vi "Add Icon From Picture.vi"(7 "Icon Index (Next)":i32=-1, 8 "error in (no error)":errorcluster, 9 "Icon Name":string, 10 "Picture":picture, 11 "Toolbar Control in":refnum<class "Toolbar Control.lvclass">) -> (0 "error out":errorcluster, 3 "Toolbar Control out":refnum<class "Toolbar Control.lvclass">)   [LabVIEW 2011, in "Toolbar Control.lvclass"]
doc: "This VI will add the image <B>Picture</B> to the <B>Toolbar Control in</B> at the available location or if specified by <B>Icon Index (Next)</B>. The name of the icon is specified by <B>Icon Name</B>.\n\n-------------\nDeveloped by Brian Hoover (hooovahh)"
uses:
  Toolbar Control.lvclass
  Toolbar Control.lvclass/Toolbar Control.ctl
  Controls/Icon Data.ctl
  <vilib>/picture/picture.llb/imagedata.ctl
  Controls/Button State.ctl
  Controls/Icon Type.ctl
  <vilib>/Utility/miscctls.llb/LVRectTypeDef.ctl
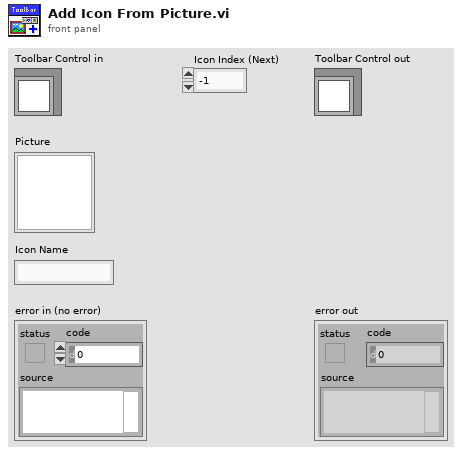
[diagram p1: front panel]
types:
  T1 = typedef "LVRectTypeDef.ctl" = cluster{"Left":i16, "Top":i16, "Right":i16, "Bottom":i16}
  T2 = typedef "Toolbar Control.lvclass/Icon Data.ctl" = cluster{"Original Image Path":path, "Original Image Data":T3, "Scaled Icon":picture, "Button Name":string, "Button State":T4, "Icon Type":T5}
  T3 = typedef "imagedata.ctl" = cluster{"image type":i32, "image depth":i32, "image":u8[], "mask":u8[], "colors":u32[], "Rectangle":cluster{"left":i16, "top":i16, "right":i16, "bottom":i16}}
  T4 = typedef "Toolbar Control.lvclass/Button State.ctl" = enum8{"Enabled", "Disabled", "Disabled and Grayed Out"}
  T5 = typedef "Icon Type.ctl" = enum16{"Normal Icon", "Separator Icon", "More Options"}
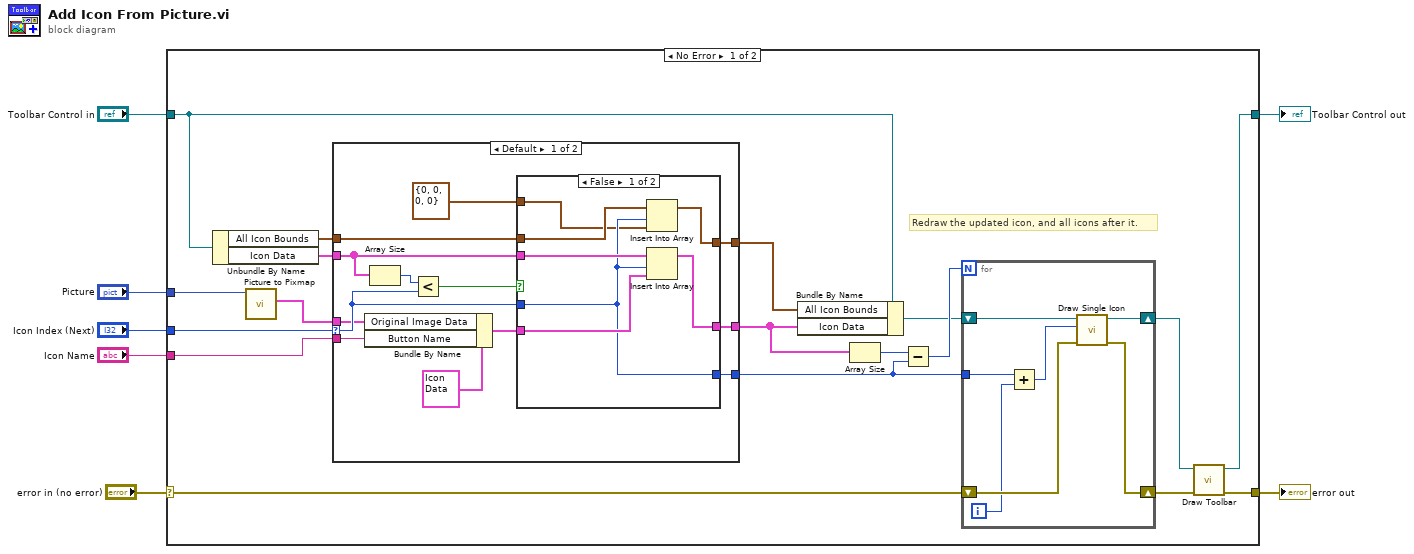
[diagram p0: block diagram]
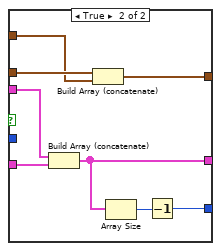
[diagram p2: hidden frame]
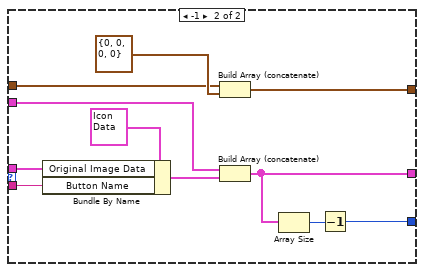
[diagram p3: hidden frame]
diagram:
  n1 = case shown="No Error" "error in (no error)" {
    selector: "error in (no error)" -> [w12 w73]
    tunnel: [w8 w73] -> w6
    tunnel: [w9 w72] -> w4
    tunnel: "Toolbar Control in" -> [w25 w72]
    tunnel: "Picture" -> [w21 _]
    tunnel: "Icon Index (Next)" -> [w23 _]
    tunnel: "Icon Name" -> [w22 _]
    frame No Error {
      # "Redraw the updated icon, and all icons after it."
      n2 = Unbundle By Name(w25) -> ("All Icon Bounds"=w19:T1[], "Icon Data"=w24:T2[])
      n3 = call <vilib>:"Picture to Pixmap.vi"("picture"=w21) -> ("image data"=w20:T3)  [unwired: 9 in, 1 out]
      n4 = case shown="Default" w23 {
        selector: w23 -> [w38 _]
        tunnel: w20 -> [w37 w70]
        tunnel: w22 -> [w45 w69]
        tunnel: w24 -> [w43 w68]
        tunnel: [w39 w65] -> w14
        tunnel: [w36 w64] -> w15
        tunnel: w19 -> [w35 w62]
        tunnel: [w34 w61] -> w18
        frame Default {
          n5 = Bundle By Name(cluster=T2 {"Original Image Path"=path "", "Original Image Data"={"image type"=0, "image depth"=0, "image"=[], "mask"=[], "colors"=[], "Rectangle"={"left"=0, "top"=0, "right"=0, "bottom"=0}}, "Scaled Icon"=bytes[0], "Button Name"="", "Button State"=enum."Enabled", "Icon Type"=enum."Normal Icon"} ("Cluster"), "Original Image Data"=w37, "Button Name"=w45) -> (w40:T2)
          n6 = Array Size(array=w43) -> (size(s)=w42:i32)
          n7 = Less?(x=w42, y=w38) -> (x < y?=w41:bool)
          n8 = case shown="False" w41 {
            tunnel: w43 -> [w52 w60]
            tunnel: w40 -> [w51 w59]
            tunnel: [w50 w57] -> w39
            tunnel: w38 -> [w47 _]
            tunnel: [w47 w56] -> w36
            tunnel: w35 -> [w48 w55]
            tunnel: [w49 w54] -> w34
            tunnel: T1 {"Left"=0, "Top"=0, "Right"=0, "Bottom"=0} ("Icon Bounds") -> [w46 w53]
            frame False {
              n9 = Insert Into Array(array=w48, index=w47, new element=w46) -> (w49:T1[])
              n10 = Insert Into Array(array=w52, index=w47, new element=w51) -> (w50:T2[])
            }
            frame True {
              n11 = Build Array (concatenate)(w60, w59) -> (w57:T2[])
              n12 = Build Array (concatenate)(w55, w53) -> (w54:T1[])
              n13 = Array Size(array=w57) -> (size(s)=w58:i32)
              n14 = Decrement(x=w58) -> (x-1=w56:i32)
            }
          }
        }
        frame -1 {
          n15 = Bundle By Name(cluster=T2 {"Original Image Path"=path "", "Original Image Data"={"image type"=0, "image depth"=0, "image"=[], "mask"=[], "colors"=[], "Rectangle"={"left"=0, "top"=0, "right"=0, "bottom"=0}}, "Scaled Icon"=bytes[0], "Button Name"="", "Button State"=enum."Enabled", "Icon Type"=enum."Normal Icon"} ("Cluster"), "Original Image Data"=w70, "Button Name"=w69) -> (w67:T2)
          n16 = Build Array (concatenate)(w62, T1 {"Left"=0, "Top"=0, "Right"=0, "Bottom"=0} ("Icon Bounds")) -> (w61:T1[])
          n17 = Build Array (concatenate)(w68, w67) -> (w65:T2[])
          n18 = Array Size(array=w65) -> (size(s)=w66:i32)
          n19 = Decrement(x=w66) -> (x-1=w64:i32)
        }
      }
      n20 = Bundle By Name(cluster=w25, "All Icon Bounds"=w18, "Icon Data"=w14) -> (w13:refnum<class "Toolbar Control.lvclass">)
      n21 = Array Size(array=w14) -> (size(s)=w17:i32)
      n22 = Subtract(x=w17, y=w15) -> (x-y=w16:i32)
      n23 = for {
        N: w16 -> [_]
        tunnel: w15 -> [w28]
        shift-right: [w31] -> w10
        shift-left: w13 -> [w32]
        shift-right: [w29] -> w11
        shift-left: w12 -> [w30]
        i -> [w27]
        n24 = Add(x=w28, y=w27) -> (x+y=w26:i32)
        n25 = call "Draw Single Icon.vi"("error in (no error)"=w30, "Icon Index"=w26, "Toolbar Control in"=w32) -> ("error out"=w29:errorcluster, "Toolbar Control out"=w31:refnum<class "Toolbar Control.lvclass">)  [unwired: 7 in]
      }
      n26 = call "Draw Toolbar.vi"("error in (no error)"=w11, "Toolbar Control in"=w10) -> ("error out"=w8:errorcluster, "Toolbar Control out"=w9:refnum<class "Toolbar Control.lvclass">)  [unwired: 7 in, 1 out]
    }
    frame Error {
    }
  }
  "error out" <- w6
  "Toolbar Control out" <- w4
